vi "TCP Engine Configuration data to Command.vi"(6 "AI":path, 9 "Serial":path, 10 "DI":path, 11 "DO":path) -> (3 "Command Data":string[](array[string]))   [LabVIEW 2024]
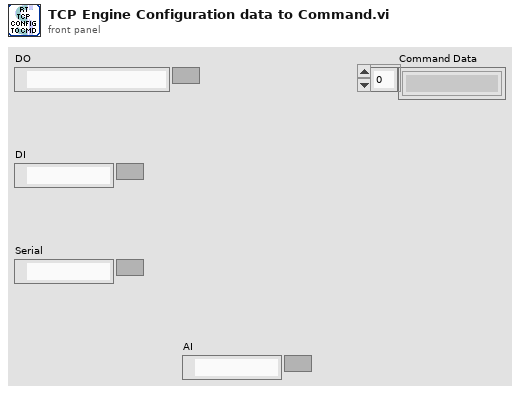
[diagram p1: front panel]
types:
  T1 = typedef "Async JSON Cluster.ctl" = cluster{"Interface":string, "Interface Data":T2}
  T2 = typedef "Async Interface Data Cluster.ctl" = cluster{"Command":string, "SubCmd":string, "Data":T3[]}
  T3 = typedef "Async Serial Configuration Cluster.ctl" = cluster{"Port":string, "Minor Frame Freq":u16, "Minor Frame Count":u16, "Frame Info":T4[], "Sensor Type":u16, "OIM Address":u16}
  T4 = typedef "Async Frame Info Cluster.ctl" = cluster{"Frame ID":u16, "Message Info":T5[]}
  T5 = typedef "Async Message Info Cluster.ctl" = cluster{"Message":u8[], "Message Name":string}
  T6 = typedef "DIO Configuration cluster.ctl" = cluster{"Interface":string, "Interface Data":T7}
  T7 = typedef "DIO Interface Data.ctl" = cluster{"Command":string, "SubCmd":string, "Frequency":u16, "Data":T8[]}
  T8 = typedef "Digital Dynamic Cluster.ctl" = cluster{"Channel":string, "Data":u8[]}
  T9 = typedef "AO JSON Data Cluster.ctl" = cluster{"Interface":string, "Interface Data":T10}
  T10 = typedef "AO Interface Data Cluster.ctl" = cluster{"Command":string, "SubCmd":string, "Data":T11[], "Timing":T12}
  T11 = typedef "AO Channel Configuration Cluster.ctl" = cluster{"Channel":string, "Min Value":dbl, "Max Value":dbl, "Type":string, "Terminal Configure":u16, "Dynamic":u8, "Dyn Type":string, "Data":dbl[], "File Name":string, "Column":i32, "Frequency":dbl}
  T12 = typedef "AO Timing Cluster.ctl" = cluster{"samples per channel":i32, "sample mode":i32, "rate":dbl}
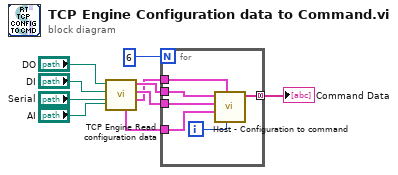
[diagram p0: block diagram]
diagram:
  n1 = call "TCP Engine Read configuration data.vi"("AI"="AI", "Serial"="Serial", "DI"="DI", "DO"="DO") -> ("Async data"=w5:T1, "DO data"=w7:T6, "DI data"=w6:T6, "AI data"=w8:T9)  [unwired: 4 in]
  n2 = for {
    N: 6 -> [_]
    tunnel: w5 -> [w16]
    tunnel: w6 -> [w15]
    tunnel: w7 -> [w14]
    tunnel: w8 -> [w13]
    tunnel: [w11] -> w10 mode=concatenating
    i -> [w12]
    n3 = call "Host - Configuration to command.vi"("Operation Index"=w12, "Async"=w16, "AI"=w13, "DO"=w14, "DI"=w15) -> ("Command Data"=w11:string[])  [unwired: 5 in, 1 out]
  }
  "Command Data" <- w10
